vi "Main.vi"(11 "Module Admin":refnum<class "Delacor_lib_QMH_Module Admin.lvclass">) -> ()   [LabVIEW 2024, in "MQTTClient.lvlib"]
doc: "This template is based from the Queued Message Handler design pattern and the Queued Message Handler Project Template that ships with LabVIEW 2014.\n\nThe main difference is that the Queue is private to this module and communication between modules is done via Broadcast and Request events.\n\nRequest events are wrapped via public API methods and are handled in the Event handler loop in this VI.\nAny module can register for Broadcast events sent by this module.\n\nThe Event Handling Loop generates messages based on user interface actions.\n\nThe Message Handling Loop processes messages generated by the Event Handling Loop, or by other messages. The messages are string values, so new messages can be added easily to the Message Cases case structure in the Message Handling Loop. Each message cluster can also provide an optional value for Message Data, which is a variant that can be converted to whatever message-specific data is required.\n_____\nBased on Delacor QMH Project Template 3.1.0.34.\n\n<b>Note:</b> This VI was modified by the <b>Validate DQMH Module</b> tool to add a call to the Error Reported VI at the end of the 'Exit' MHL frame.\n\n<b>Note:</b> This VI was modified by the <b>Validate DQMH Module</b> tool to call the Release Message Queue VI in the top-level Error case.\n\n<b>Note:</b> This VI was modified by the <b>Validate DQMH Module</b> tool to wrap the FP.Open method in the module close code with a Conditional Disable Structure so it does not execute when the Main VI is running as a built EXE."
uses:
  MQTTClient.lvlib
  <vilib>/Delacor/Delacor QMH/Libraries/Module Admin_class/Delacor_lib_QMH_Module Admin.lvclass
  <vilib>/MGI/Panel Manager/Panel/Panel/Panel.lvclass
  <vilib>/Utility/miscctls.llb/LVPointTypeDef.ctl
  <vilib>/LabVIEW Open Source Project/MQTT Connection/MQTT_Base/Base Class/Public Events -- cluster.ctl
  <vilib>/LabVIEW Open Source Project/MQTT Control Packets/Control Packets/PUBLISH/PUBLISH.lvclass
  C:/Program Files/National Instruments/LabVIEW 2025/vi.lib/LabVIEW Open Source Project/MQTT Control Packets/Control Packets/ControlPacket/ControlPacket.lvclass
  <vilib>/LabVIEW Open Source Project/MQTT Client/Client class/Public Events -- cluster.ctl
  <vilib>/LabVIEW Open Source Project/MQTT Control Packets/Control Packets/CONNACK/Connect Return Code -- enum.ctl
  Module Data--cluster.ctl
  <vilib>/LabVIEW Open Source Project/MQTT Client/Client class/Client.lvclass
  C:/Program Files/National Instruments/LabVIEW 2025/vi.lib/LabVIEW Open Source Project/MQTT Connection/MQTT_Base/Base Class/MQTT_Base.lvclass
  MQTT Configuration--cluster.ctl
  <vilib>/Delacor/Delacor QMH/Libraries/Message Queue_class/Delacor_lib_QMH_Message Queue.lvclass/Delacor_lib_QMH_Message Queue.ctl
  Stop Argument--cluster.ctl
  <vilib>/Delacor/Delacor QMH/Libraries/Module Admin_class/Delacor_lib_QMH_Module Admin.lvclass/Delacor_lib_QMH_Module Admin.ctl
  Initialise Connection Argument--cluster.ctl
  Ping Connection Argument--cluster.ctl
  Publish to MQTT Topic Argument--cluster.ctl
  Close Connection Argument--cluster.ctl
  Connect to MQTT Server Argument--cluster.ctl
  Sleep Ping Helper Loop Argument--cluster.ctl
  Subscribe to MQTT Topic Argument--cluster.ctl
  Launch Argument--cluster.ctl
  <vilib>/LabVIEW Open Source Project/MQTT Control Packets/Control Packets/ControlPacket/ControlPacket.lvclass/ControlPacket.ctl
  <vilib>/Delacor/Delacor QMH/Libraries/Message Queue_class/Delacor_lib_QMH_Enqueue Message (Single).vi
  <vilib>/Delacor/Delacor QMH/Libraries/Module Admin_class/Delacor_lib_QMH_Get External Launch.vi
  <vilib>/Utility/error.llb/Error Cluster From Error Code.vi
  <vilib>/ErrorRing/Error Ring.xnode
  <vilib>/Delacor/Delacor QMH/Libraries/Message Queue_class/Delacor_lib_QMH_Message Queue.lvclass
  <vilib>/MGI/Panel Manager/Panel/Panel Helper/Panel Helper.lvclass
  <vilib>/LabVIEW Open Source Project/MQTT Connection/MQTT_Base/Base Class/MQTT_Base.lvclass
  <vilib>/LabVIEW Open Source Project/MQTT Control Packets/Control Packets/ControlPacket/ControlPacket.lvclass
  <vilib>/LabVIEW Open Source Project/MQTT Control Packets/Control Packets/CONNACK/CONNACK.lvclass
panel:
  out "Published":bool
  out "connected":bool
  out "Server responded":bool
  in  "Panel":refnum<class "Panel.lvclass">
  in  "Simulate MHL Error":bool
  in  "Simulate EHL Error":bool
  out "error out":errorcluster
  out "Status":string
  # "This is a template that creates a DQMH Singleton using the MGI Panel Manager Framwork.\n\nImplement your user interface on this front panel. The Panel Manager Framework will manage showing and hiding the panel in the appropriate spot. \n\nSee the block diagram for more information on how to use this template."
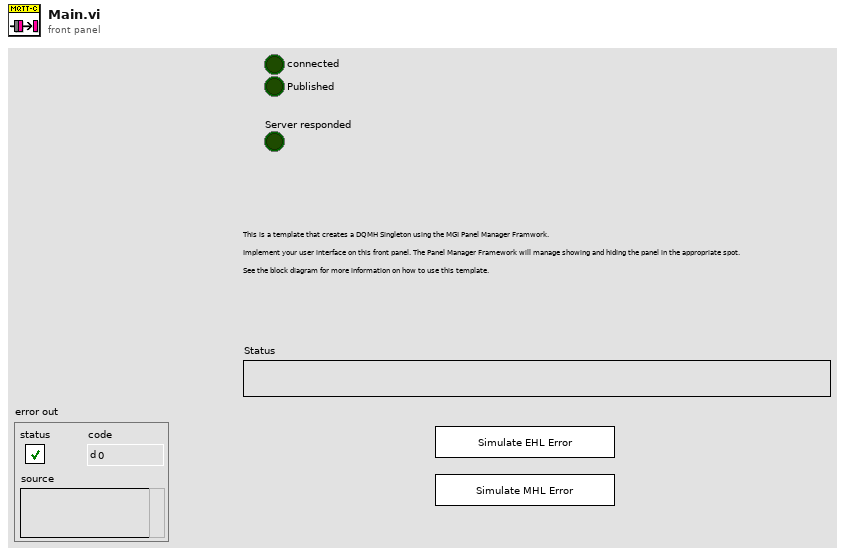
[diagram p1: front panel]
types:
  T1 = typedef "MQTT Client.lvlib/Client.lvclass/Public Events -- cluster.ctl" = cluster{"Connection Status":refnum<user-event>, "Connected":refnum<user-event>, "Application Message":refnum<user-event>}
  T2 = typedef "MQTT Base.lvlib/MQTT_Base.lvclass/Public Events -- cluster.ctl" = cluster{"Stop Event":refnum<user-event>, "Error Event":refnum<user-event>, "Inbound Message":refnum<user-event>}
  T3 = typedef "LVPointTypeDef.ctl" = cluster{"Horizontal":i16, "Vertical":i16}
  T4 = typedef "MQTTClient.lvlib/Request Events--cluster.ctl" = cluster{"Stop Module":refnum<user-event>, "Show Panel":refnum<user-event>, "Hide Panel":refnum<user-event>, "Get Module Execution Status":refnum<user-event>, "Show Diagram":refnum<user-event>, "Change Panel":refnum<user-event>, "Initialise Connection":refnum<user-event>, "Ping Connection":refnum<user-event>, "Publish to MQTT Topic":refnum<user-event>, "Close Connection":refnum<user-event>, "Connect to MQTT Server":refnum<user-event>, "Private":cluster{"Reset Ping Helper Loop Timeout":refnum<user-event>, "Sleep Ping Helper Loop":refnum<user-event>, "Register MQTT Client Events":refnum<user-event>}, "Subscribe to MQTT Topic":refnum<user-event>, "Launch":refnum<user-event>, "Private.Wake Connection Helper Loop":refnum<user-event>}
  T5 = typedef "Panel.lvlib/Panel Helper.lvclass/Panel Events.ctl" = cluster{"My Panel":refnum<user-event>, "Top Level Initialized":refnum<user-event>}
  T6 = typedef "MQTTClient.lvlib/Module Data--cluster.ctl" = cluster{"Status":string, "MQTT_Base":refnum<class "Client.lvclass">, "Published Values":map{string, string}, "Configuration":T7, "Subscribed Values":map{string, string}}
  T7 = typedef "MQTTClient.lvlib/MQTT Configuration--cluster.ctl" = cluster{"Client-ID":string, "Server Address":string, "Server Port":u16}
  T8 = typedef "MQTTClient.lvlib/Stop Argument--cluster.ctl" = cluster{"Origin":string, "Exit via Stop Module Req?":bool, "Wait for Module to stop?":bool}
  T9 = typedef "MQTTClient.lvlib/Initialise Connection Argument--cluster.ctl" = cluster{"Client ID":string, "Server Address":string, "Server Port":u16}
  T10 = typedef "MQTTClient.lvlib/Ping Connection Argument--cluster.ctl" = cluster{"Boolean":bool}
  T11 = typedef "MQTTClient.lvlib/Publish to MQTT Topic Argument--cluster.ctl" = cluster{"Topic":string, "Value":string}
  T12 = typedef "MQTTClient.lvlib/Close Connection Argument--cluster.ctl" = cluster{"Boolean":bool}
  T13 = typedef "MQTTClient.lvlib/Connect to MQTT Server Argument--cluster.ctl" = cluster{"Boolean":bool}
  T14 = typedef "MQTTClient.lvlib/Sleep Ping Helper Loop Argument--cluster.ctl" = cluster{"Boolean":bool}
  T15 = typedef "MQTTClient.lvlib/Subscribe to MQTT Topic Argument--cluster.ctl" = cluster{"Topic":string}
  T16 = typedef "MQTTClient.lvlib/Launch Argument--cluster.ctl" = cluster{"Boolean":bool}
  T17 = enum32{"invalid lock state", "Not Locked", "Locked (No Password)", "Password-protected"}
  T18 = typedef "MQTTClient.lvlib/Config--cluster.ctl" = cluster{"Client-ID":string, "Server Address":string, "Server Port":u16}
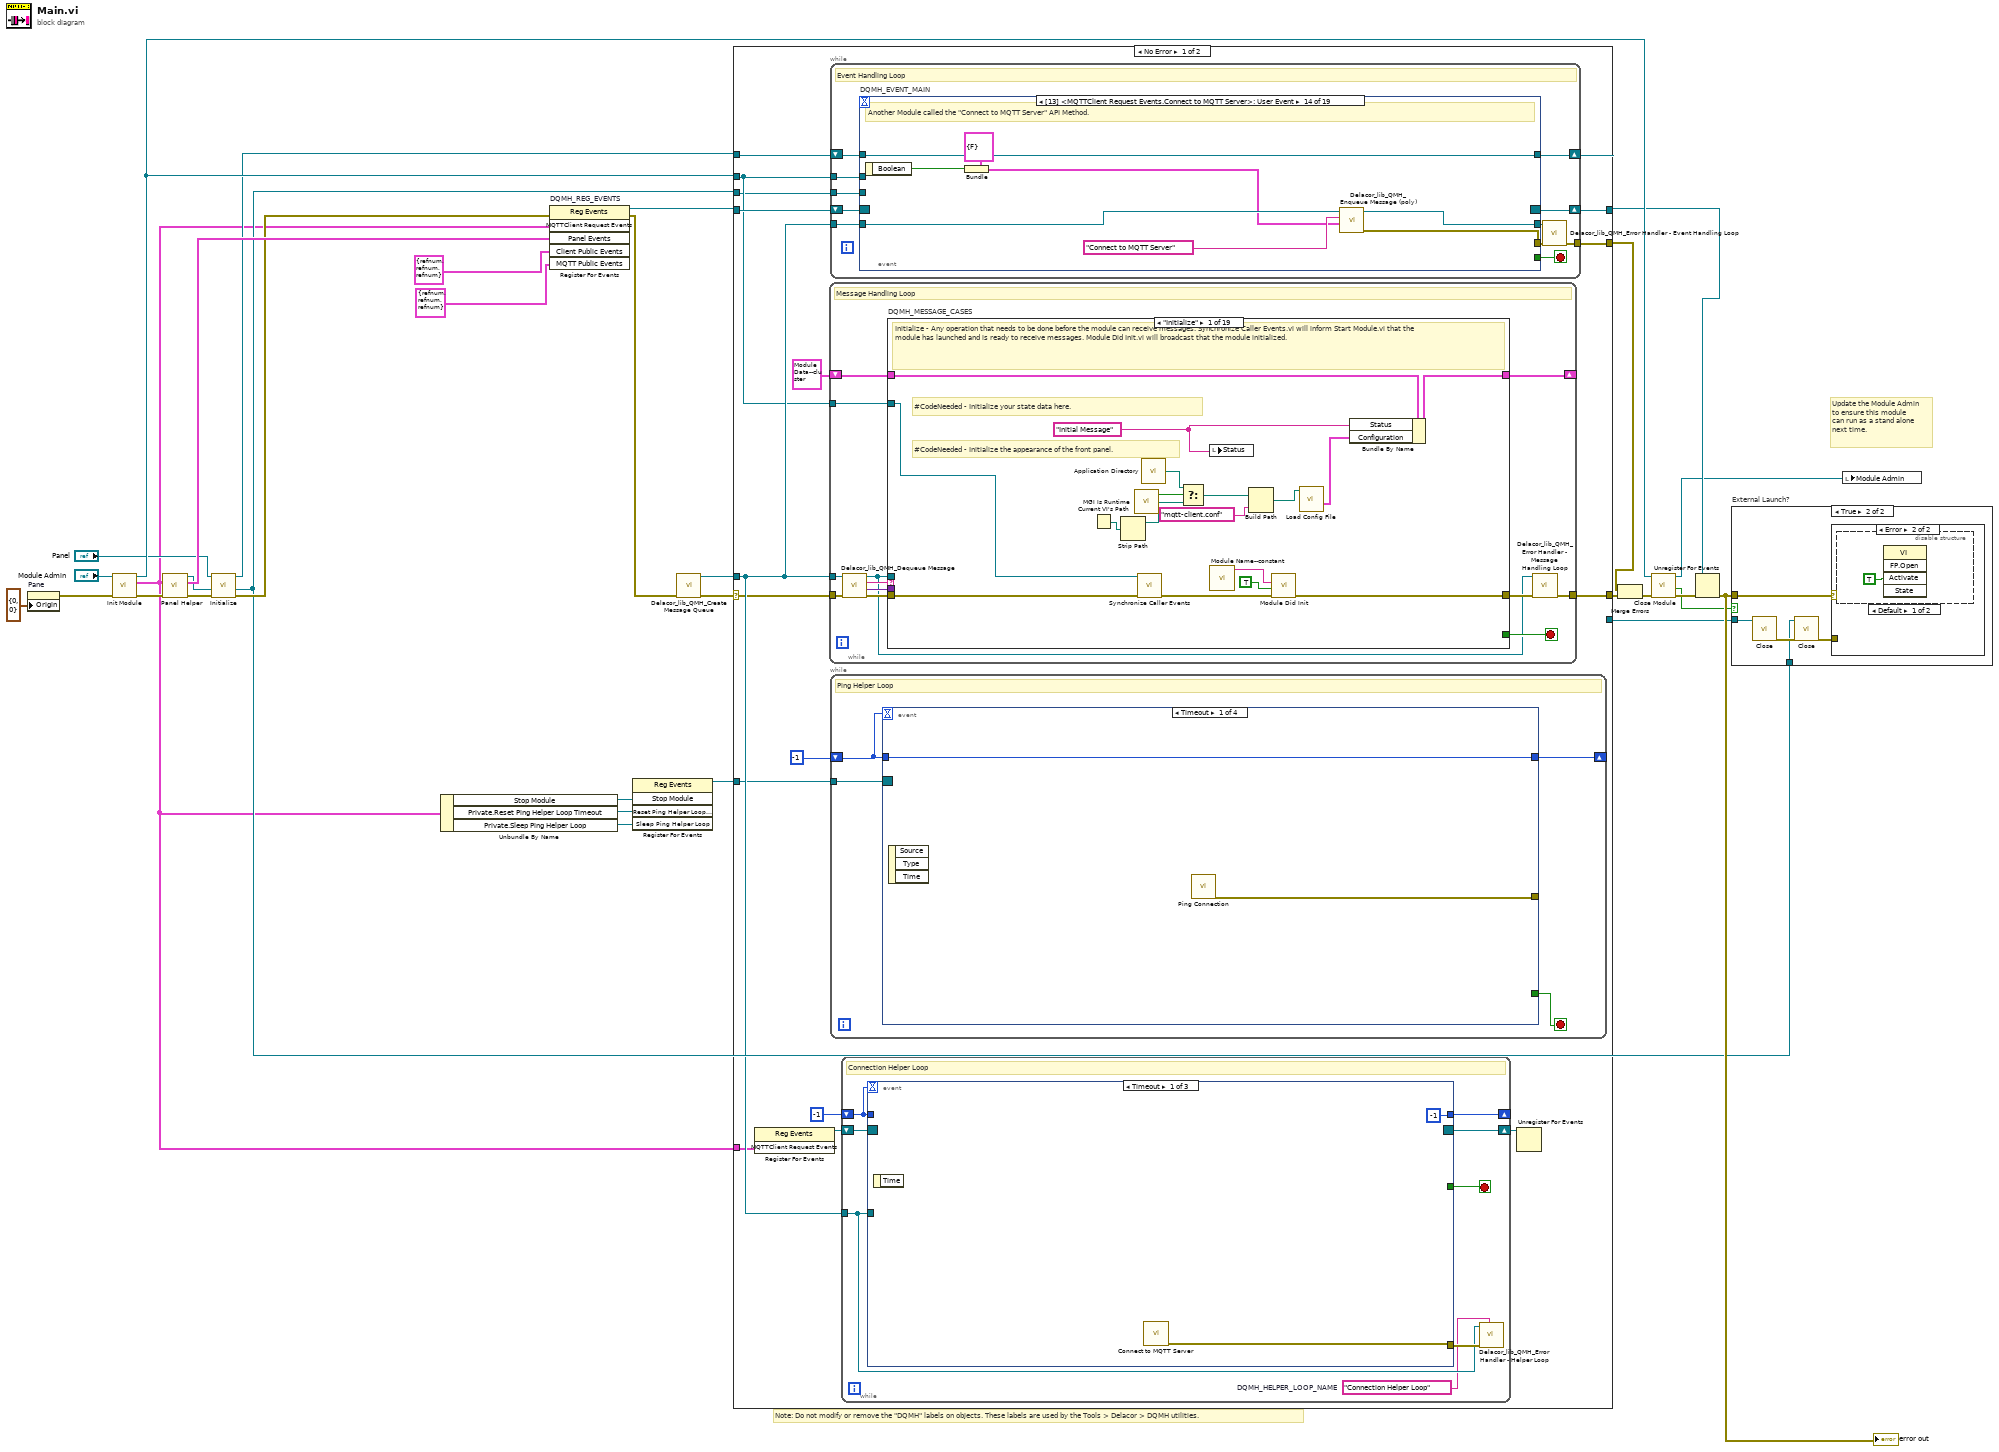
[diagram p0: block diagram]
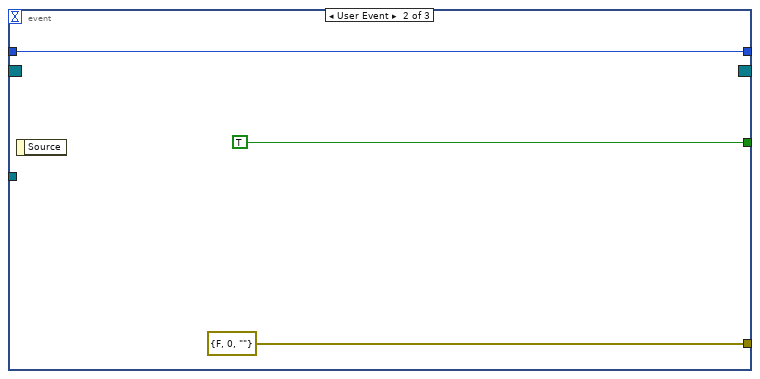
[diagram p5: hidden frame]
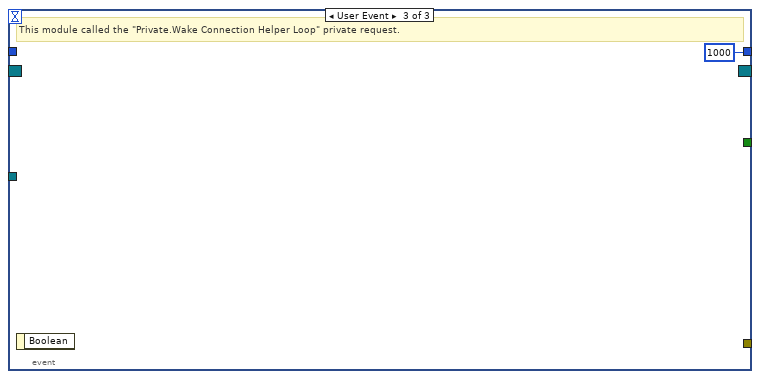
[diagram p6: hidden frame]
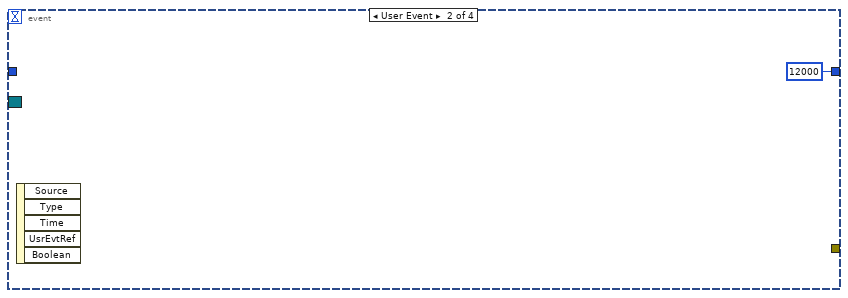
[diagram p7: hidden frame]
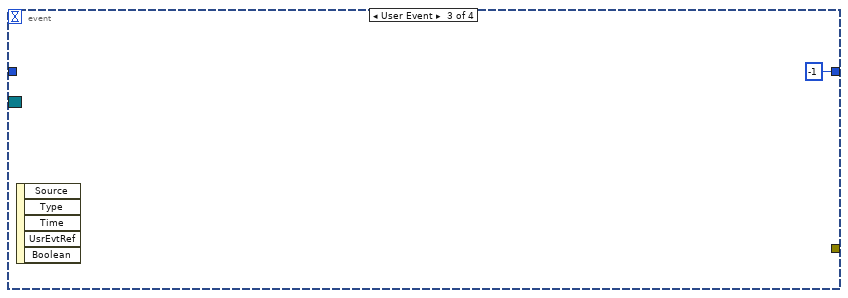
[diagram p8: hidden frame]
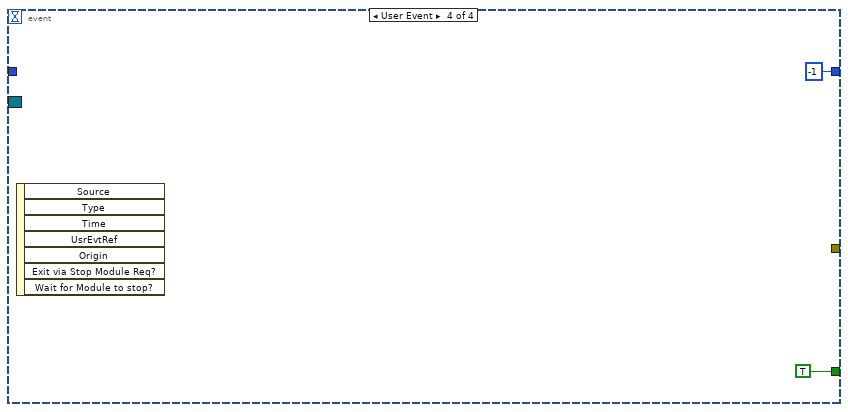
[diagram p9: hidden frame]
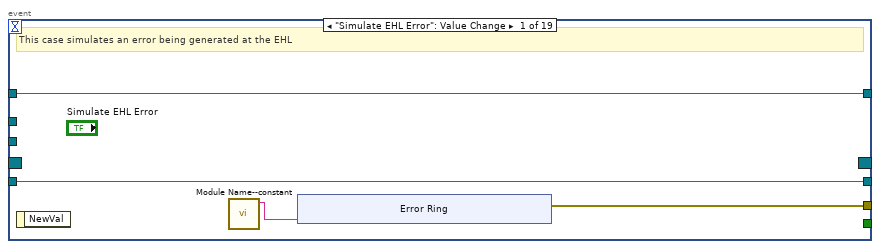
[diagram p10: hidden frame]
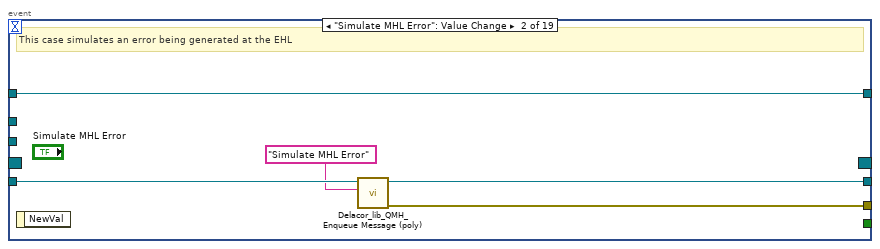
[diagram p11: hidden frame]
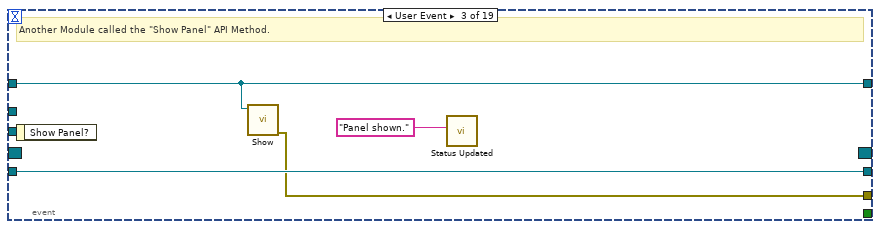
[diagram p12: hidden frame]
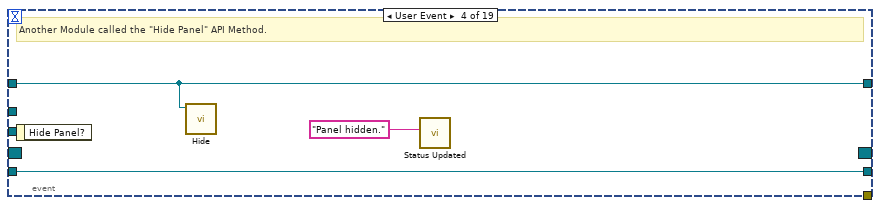
[diagram p13: hidden frame]
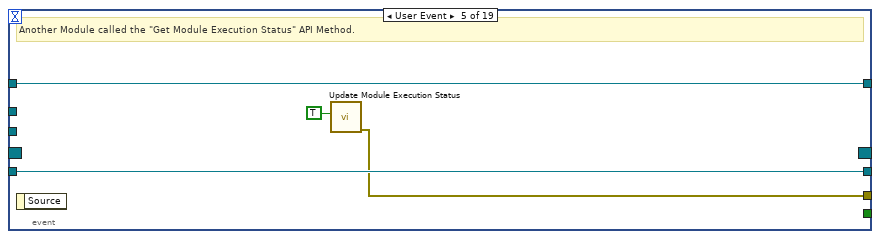
[diagram p14: hidden frame]
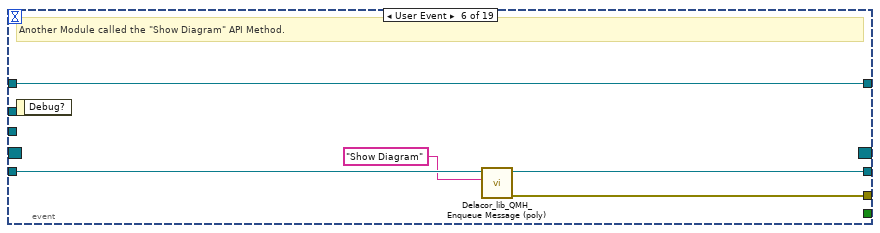
[diagram p15: hidden frame]
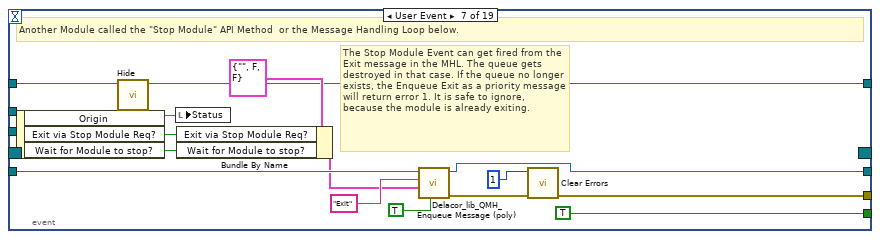
[diagram p16: hidden frame]
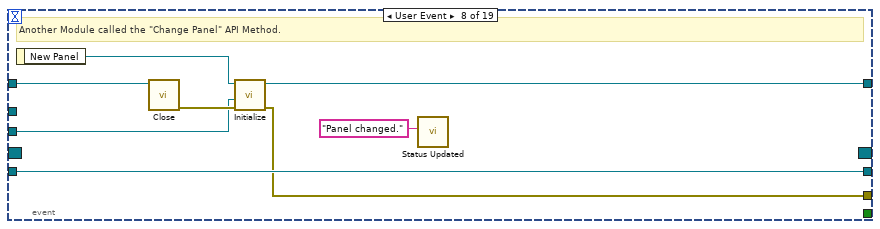
[diagram p17: hidden frame]
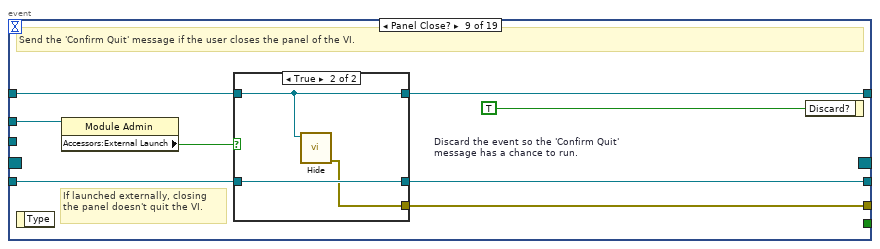
[diagram p18: hidden frame]
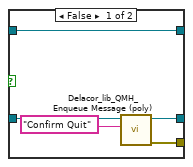
[diagram p19: hidden frame]
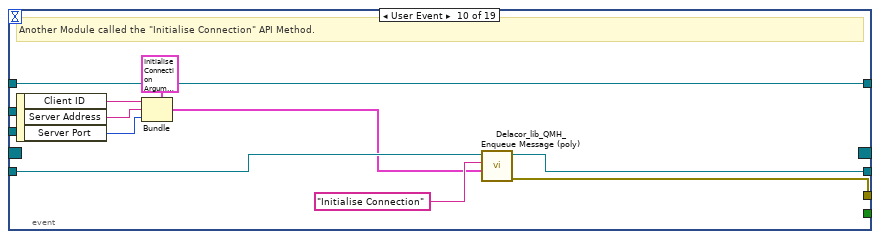
[diagram p20: hidden frame]
diagram:
  # "Note: Do not modify or remove the \"DQMH\" labels on objects. These labels are used by the Tools > Delacor > DQMH utilities."
  # "Update the Module Admin to ensure this module can run as a stand alone next time."
  n1 = property on="Pane" class="Pane"("Origin"=T3 {"Horizontal"=0, "Vertical"=0}) -> (error out=w8:errorcluster)  [unwired: 2 in, 1 out]
  n2 = call "Init Module.vi"("error in (no error)"=w8, "Singleton Module Admin in"="Module Admin") -> ("error out"=w18:errorcluster, "MQTTClient Request Events"=w1:T4, "Singleton Module Admin out"=w32:refnum<class "Delacor_lib_QMH_Module Admin.lvclass">)  [unwired: 7 in]
  n3 = call <vilib>:"Panel Helper.vi"("Error In"=w18) -> ("Error Out"=w15:errorcluster, "Panel Events"=w17:T5, "Panel Helper out"=w14:refnum<class "Panel Helper.lvclass">)  [unwired: 8 in]
  n4 = call <vilib>:"Initialize.vi"("error in (no error)"=w15, "My Helper in"=w14, "Panel In"="Panel") -> ("error out"=w12:errorcluster, "My Helper out"=w11:refnum<class "Panel Helper.lvclass">, "Panel Out"=w10:refnum<class "Panel.lvclass">)  [unwired: 6 in]
  n5 = Unbundle By Name(w1) -> ("Stop Module"=w5:refnum<user-event>, "Private.Reset Ping Helper Loop Timeout"=w6:refnum<user-event>, "Private.Sleep Ping Helper Loop"=w7:refnum<user-event>)
  n6 = register-events "DQMH_REG_EVENTS"(error in=w12, w1, w17, T1 {"Connection Status"=refnum, "Connected"=refnum, "Application Message"=refnum} ("Client Public Events"), T2 {"Stop Event"=refnum, "Error Event"=refnum, "Inbound Message"=refnum} ("MQTT Public Events")) -> (reference out=w29:refnum<event-registration>, error out=w16:errorcluster)  [unwired: 1 in]
  n7 = register-events(w5, w6, w7) -> (reference out=w4:refnum<event-registration>)  [unwired: 2 in, 1 out]
  n8 = call <vilib>:"Delacor_lib_QMH_Create Message Queue.vi"("error in"=w16) -> ("error out"=w20:errorcluster, "Message Queue"=w28:refnum<class "Delacor_lib_QMH_Message Queue.lvclass">)  [unwired: 9 in]
  n9 = case shown="No Error" w20 {
    selector: w20 -> [w43 w511]
    tunnel: [w49 w511] -> w31
    tunnel: [w48 w516] -> w30
    tunnel: w29 -> [w46 w516]
    tunnel: w28 -> [w45 w507]
    tunnel: [w44 _] -> w24
    tunnel: w32 -> [w42 w512]
    tunnel: w10 -> [w40 w508]
    tunnel: w11 -> [w41 _]
    tunnel: [w39 w508] -> w19
    tunnel: w4 -> [w38 _]
    tunnel: w1 -> [w36 _]
    frame No Error {
      n10 = register-events ("DQMH_HELPER_REGFOREVENTS")(w36) -> (reference out=w34:refnum<event-registration>)  [unwired: 2 in, 1 out]
      n11 = while {
        tunnel: w45 -> [w237]
        shift-right: [w243] -> _
        shift-left: T6 {"Status"="", "MQTT_Base"=refnum, "Published Values"={}, "Configuration"={"Client-ID"="", "Server Address"="", "Server Port"=0}, "Subscribed Values"={}} ("Data Cluster") -> [w244]
        tunnel: w43 -> [w241]
        tunnel: [w235] -> w49
        tunnel: w42 -> [w234]
        stop <- w242 stop-if-true
        # "Message Handling Loop"
        n12 = call-dynamic "Delacor_lib_QMH_Dequeue Message.vi"("error in"=w241, "Message Queue in"=w237) -> ("error out"=w240:errorcluster, "Message Data"=w238:variant, "Message"=w239:string, "Message Queue out"=w236:refnum<class "Delacor_lib_QMH_Message Queue.lvclass">)  [unwired: 6 in]
        n13 = case "DQMH_MESSAGE_CASES" shown="\"Initialize\"" w239 {
          selector: w239 -> [_ _ _ _ _ _ _ _ _ _ _ _ _ _ _ _ _ _ w496]
          tunnel: w236 -> [_ _ _ _ _ _ _ _ _ _ _ _ _ _ _ w460 w475 w492 _]
          tunnel: w240 -> [w256 w268 w272 w290 w306 w320 w358 w380 w400 w415 w428 w438 w441 w444 w449 w466 w479 w494 _]
          tunnel: [w257 w269 w271 w288 w298 w308 w349 w376 w390 w403 w425 w435 w439 w442 w447 w457 w477 w488 w497] -> w245
          tunnel: w244 -> [w262 w270 w273 w289 w292 w312 w354 w369 w394 w407 w417 w432 w440 w443 w448 w465 w478 w491 w498]
          tunnel: [w261 w270 w273 w289 w302 w311 w353 w368 w393 w406 w416 w432 w440 w443 w448 w465 w478 w491 w498] -> w243
          tunnel: [_ _ _ _ _ _ _ _ _ _ _ _ _ _ _ _ _ w490 _] -> w242
          tunnel: w238 -> [_ w267 _ _ w305 w319 w357 w379 w399 w413 w427 w437 _ _ _ w464 _ w487 _]
          tunnel: w234 -> [w254 _ _ _ _ _ _ _ _ _ _ _ _ _ _ w459 _ w481 _]
          frame "Initialize" {
            w260 = "Initial Message" ("Initial Message")
            # "#CodeNeeded - Initialize the appearance of the front panel."
            # "#CodeNeeded - Initialize your state data here."
            # "Initialize - Any operation that needs to be done before the module can receive messages. Synchronize Caller Events.vi will inform Start Module.vi that the module has launched and is ready to receive messages. Module Did Init.vi will broadcast that the module initialized."
            n14 = Current VI's Path() -> (path=w247:path)
            n15 = Strip Path(path=w247) -> (stripped path=w246:path)  [unwired: 1 out]
            n16 = call <userlib>:"MGI Is Runtime.vi"() -> ("Run Time System?"=w250:bool)  [unwired: 7 in]
            n17 = call "Synchronize Caller Events.vi"("error in (no error)"=w256, "Singleton Module Admin in"=w254) -> ("error out"=w255:errorcluster)  [unwired: 8 in, 1 out]
            n18 = call <vilib>:"Application Directory.vi"() -> ("Application Directory"=w249:path)
            n19 = Select(t=w249, s=w250, f=w246) -> (s? t:f=w248:path)
            n20 = local write "Status"(w260) -> ()
            n21 = call "Module Name--constant.vi"() -> ("Module Name"=w258:string)  [unwired: 11 in]
            n22 = Build Path(base path=w248, name or relative path="mqtt-client.conf") -> (appended path=w252:path)
            n23 = call "Module Did Init.vi"("error in (no error)"=w255, "Initialized?"=TRUE, "Origin"=w258) -> ("error out"=w257:errorcluster)  [unwired: 8 in]
            n24 = call "Load Config File.vi"("File Path"=w252) -> ("value"=w251:T18)  [unwired: 10 in]
            n25 = Bundle By Name(cluster=w262, "Status"=w260, "Configuration"=w251) -> (w261:T6)
          }
          frame "Update Display" {
            # "Broadcast updated status to any VI registered to listen to this module's broadcast events."
            # "Convert the message data to a string to display in the Status indicator."
            # "#CodeRecommended - If you wish to decouple the Message Handling Loop from your user interface, consider creating User Events (like the \"Stop\" event in this VI) to message the Event Handling Loop whenever the user interface needs updating."
            # "Update Display - Update user interface here."
            n26 = Variant To Data(error in=w268, type="" ("Empty String Constant"), Variant=w267) -> (data=w265:string, error out=w264:errorcluster)
            "Status" <- w265
            n27 = call "Status Updated.vi"("error in (no error)"=w264, "Status"=w265) -> ("error out"=w263:errorcluster)  [unwired: 9 in]
            n28 = Merge Errors(w263) -> (w269:errorcluster)
          }
          frame "Show Diagram" {
            # "Show Diagram - Show the block diagram of this VI. Used as a debugging tool. There is a button in the module tester that fires the Show Diagram request, which runs this message. Note that the diagram will not be displayed if it is password-protected and the password is not in the cache."
            n29 = disable-structure shown="RUN_TIME_ENGINE==False" {
              disable-tunnel: [w281 w287] -> w271
              disable-tunnel: w272 -> [w280 w287]
              frame condition #0 (active) {
                # "functionality not available in exe"
                n30 = invoke class="VI" method="Lock State.Get"(error in=w280) -> (error out=w279:errorcluster, "Get Lock State"=w278:T17, "pwd in cache"=w275:bool)  [unwired: 3 in, 1 out]
                n31 = Equal?(x=T17."Password-protected", y=w278) -> (x = y?=w276:bool)
                n32 = Compound Arithmetic op=AND(w276, invert w275) -> (w274:bool)
                n33 = case shown="False" w274 {
                  tunnel: [w284 w286] -> w281
                  tunnel: w279 -> [w282 w286]
                  frame False {
                    n34 = property class="VI"(error in=w282, "BDWin.Open"=TRUE ("Block Diagram Window:Open")) -> (error out=w284:errorcluster)  [unwired: 1 in, 1 out]
                    n35 = call "Status Updated.vi"("Status"="Block Diagram shown." ("format string")) -> ()  [unwired: 10 in, 1 out]
                  }
                  frame True {
                    # "Password-protected VI, and the password is not in the cache. Do not show the diagram."
                  }
                }
              }
              frame condition #1 {
              }
            }
          }
          frame "--- Module Specific ---" {
            # "Separator -- The following cases handle messages specific to this Module."
            n36 = Merge Errors(w290) -> (w288:errorcluster)
          }
          frame "Initialise Connection" {
            # "Initialises a connection to the MQTT broker."
            n37 = Variant To Data(error in=w306, type=T9 {"Client ID"="BTSCLIENT-001", "Server Address"="localhost", "Server Port"=1883} ("Initialise Connection Argument"), Variant=w305) -> (data=w303:T9)  [unwired: 1 out]
            n38 = Unbundle By Name(w292) -> ("MQTT_Base"=w296:refnum<class "Client.lvclass">)
            n39 = Unbundle By Name(w303) -> ("Client ID"=w301:string, "Server Address"=w299:string, "Server Port"=w300:u16)
            n40 = call <vilib>:"Stop.vi"("MQTT_Base in"=w296) -> ("error out"=w294:errorcluster, "MQTT_Base out"=w295:refnum<class "Client.lvclass">)  [unwired: 8 in, 1 out]
            n41 = call <vilib>:"Destroy.vi"("error in (no error)"=w294, "MQTT_Base in"=w295) -> ("error out"=w293:errorcluster)  [unwired: 8 in, 1 out]
            n42 = call <vilib>:"Clear Errors.vi"("error in (no error)"=w293) -> ("error out"=w291:errorcluster)  [unwired: 5 in, 1 out]
            n43 = call "Initialise Connection--SubVI.vi"("Client ID"=w301, "error in (no error)"=w291, "remote port (1883)"=w300, "address (localhost)"=w299) -> ("error out"=w298:errorcluster, "MQTT_Base out"=w297:refnum<class "Client.lvclass">)  [unwired: 6 in]
            n44 = Bundle By Name(cluster=w292, "Configuration.Client-ID"=w301, "Configuration.Server Address"=w299, "Configuration.Server Port"=w300, "MQTT_Base"=w297) -> (w302:T6)
          }
          frame "Connect to MQTT Server" {
            # "Connects to MQTT server."
            n45 = Variant To Data(error in=w320, type=T13 {"Boolean"=FALSE} ("Connect to MQTT Server Argument"), Variant=w319) -> (error out=w310:errorcluster)  [unwired: 1 out]
            n46 = Unbundle By Name(w312) -> ("MQTT_Base"=w315:refnum<class "Client.lvclass">)
            n47 = call <vilib>:"isConnected.vi"("error in (no error)"=w310, "Client in"=w315) -> ("error out"=w317:errorcluster, "connected"=w313:bool, "Client out"=w316:refnum<class "Client.lvclass">)  [unwired: 7 in]
            n48 = case shown="False" w313 {
              selector: w313 -> [_ w345]
              tunnel: w317 -> [w336 w346]
              tunnel: w316 -> [w335 w347]
              tunnel: [w330 w346] -> w309
              tunnel: [w333 w347] -> w314
              tunnel: [w331 w345] -> w307
              frame False {
                # "Connect"
                n49 = call <vilib>:"Connect to Server.vi"("timeout (2000 ms)"=2000, "Keep Alive (s)"=u16 60, "error in (no error)"=w336, "Client in"=w335) -> ("error out"=w332:errorcluster, "timed out"=w328:bool, "Client out"=w334:refnum<class "Client.lvclass">)  [unwired: 4 in, 1 out]
                n50 = case shown="True" w328 {
                  tunnel: w334 -> [w341 w344]
                  tunnel: [w340 w344] -> w333
                  tunnel: w332 -> [w339 w343]
                  tunnel: [w338 FALSE ("connected")] -> w331
                  tunnel: [w337 w343] -> w330
                  frame False {
                    n51 = call <vilib>:"isConnected.vi"("error in (no error)"=w339, "Client in"=w341) -> ("error out"=w337:errorcluster, "connected"=w338:bool, "Client out"=w340:refnum<class "Client.lvclass">)  [unwired: 7 in]
                  }
                  frame True {
                  }
                }
              }
              frame True {
                # "Already Connected"
              }
            }
            "connected" <- w307
            n52 = Bundle By Name(cluster=w312, "MQTT_Base"=w314) -> (w311:T6)
            n53 = case shown="False" w307 {
              tunnel: w309 -> [w322 w326]
              tunnel: [w321 w324] -> w308
              frame False {
                n54 = call "Wake Connection Helper Loop.vi"() -> ("error out"=w323:errorcluster)  [unwired: 11 in]
                n55 = Merge Errors(w323, w322) -> (w321:errorcluster)
              }
              frame True {
                n56 = call "Reset Ping Helper Loop Timeout.vi"() -> ("error out"=w325:errorcluster)  [unwired: 11 in]
                n57 = Merge Errors(w325, w326) -> (w324:errorcluster)
              }
            }
          }
          frame "Ping Connection" {
            # "Pings the MQTT broker."
            n58 = Variant To Data(error in=w358, type=T10 {"Boolean"=FALSE} ("Ping Connection Argument"), Variant=w357) -> (error out=w351:errorcluster)  [unwired: 1 out]
            n59 = Unbundle By Name(w354) -> ("MQTT_Base"=w355:refnum<class "Client.lvclass">)
            n60 = call <vilib>:"Ping.vi"("error in (no error)"=w351, "Client in"=w355) -> ("error out"=w350:errorcluster, "Server responded"=w348:bool, "Client out"=w352:refnum<class "Client.lvclass">)  [unwired: 6 in, 1 out]
            "Server responded" <- w348
            n61 = Bundle By Name(cluster=w354, "MQTT_Base"=w352) -> (w353:T6)
            n62 = case shown="False" w348 {
              tunnel: w350 -> [w360 w363]
              tunnel: [w359 w362] -> w349
              frame False {
                n63 = call "Wake Connection Helper Loop.vi"() -> ("error out"=w361:errorcluster)  [unwired: 11 in]
                n64 = Merge Errors(w361, w360) -> (w359:errorcluster)
              }
              frame True {
                n65 = call "Reset Ping Helper Loop Timeout.vi"() -> ("error out"=w364:errorcluster)  [unwired: 11 in]
                n66 = Merge Errors(w364, w363) -> (w362:errorcluster)
              }
            }
          }
          frame "Publish to MQTT Topic" {
            # "Publishes to a MQTT topic."
            n67 = Variant To Data(error in=w380, type=T11 {"Topic"="", "Value"=""} ("Publish to MQTT Topic Argument"), Variant=w379) -> (data=w377:T11, error out=w366:errorcluster)
            n68 = Unbundle By Name(w377) -> ("Topic"=w370:string, "Value"=w367:string)
            n69 = String To Byte Array(string=w367) -> (unsigned byte array=w373:u8[])
            n70 = Unbundle By Name(w369) -> ("MQTT_Base"=w375:refnum<class "Client.lvclass">)
            n71 = call <vilib>:"Publish (Raw Payload).vi"("error in (no error)"=w366, "Binary Payload"=w373, "Topic Name"=w370, "Client in"=w375) -> ("error out"=w365:errorcluster, "Published"=w371:bool, "Client out"=w374:refnum<class "Client.lvclass">)  [unwired: 5 in]
            "Published" <- w371
            n72 = Bundle By Name(cluster=w369, "MQTT_Base"=w374) -> (w372:T6)
            n73 = case shown="True" w371 {
              tunnel: w372 -> [w386 w389]
              tunnel: w370 -> [w387 _]
              tunnel: [w384 w389] -> w368
              frame False {
                # "If publish fails remove record of last published value"
                n74 = Unbundle By Name(w386) -> ("Published Values"=w388:map{string, string})
                n75 = Remove From Map(10:w387, 11:w388) -> (3:w385:map{string, string})  [unwired: 2 out]
                n76 = Bundle By Name(cluster=w386, "Published Values"=w385) -> (w384:T6)
              }
              frame True {
              }
            }
            n77 = flat-sequence {
              tunnel: [w382] -> w376
              tunnel: w365 -> [w381]
              frame #0 {
                n78 = call "Reset Ping Helper Loop Timeout.vi"() -> ("error out"=w383:errorcluster)  [unwired: 11 in]
                n79 = Merge Errors(w383, w381) -> (w382:errorcluster)
              }
            }
          }
          frame "Subscribe to MQTT Topic" {
            # "Subscribes to an MQTT topic."
            n80 = Variant To Data(error in=w400, type=T15 {"Topic"=""} ("Subscribe to MQTT Topic Argument"), Variant=w399) -> (data=w397:T15, error out=w391:errorcluster)
            n81 = Unbundle By Name(w397) -> ("Topic"=w396:string)
            n82 = Unbundle By Name(w394) -> ("MQTT_Base"=w395:refnum<class "Client.lvclass">)
            n83 = call <vilib>:"Subscribe (Scalar).vi"("error in (no error)"=w391, "Topic Filter"=w396, "Client in"=w395) -> ("error out"=w390:errorcluster, "Client out"=w392:refnum<class "Client.lvclass">)  [unwired: 6 in, 1 out]
            n84 = Bundle By Name(cluster=w394, "MQTT_Base"=w392) -> (w393:T6)
          }
          frame "Handle PUBLISH Data" {
            n85 = Variant To Data(error in=w415, type=refnum<class "PUBLISH.lvclass"> refnum ("PUBLISH"), Variant=w413) -> (data=w410:refnum<class "PUBLISH.lvclass">, error out=w411:errorcluster)
            n86 = Unbundle By Name(w407) -> ("Subscribed Values"=w408:map{string, string})
            n87 = call <vilib>:"getTopicName.vi"("error in (no error)"=w411, "PUBLISH in"=w410) -> ("error out"=w404:errorcluster, "Topic"=w402:string, "PUBLISH out"=w409:refnum<class "PUBLISH.lvclass">)  [unwired: 7 in]
            n88 = call <vilib>:"Read Payload.vi"("ControlPacket in"=w409) -> ("Payload"=w412:u8[])  [unwired: 9 in, 1 out]
            n89 = Byte Array To String(unsigned byte array=w412) -> (string=w401:string)
            n90 = Insert Into Map(map in=w408, key=w402, value=w401) -> (map out=w405:map{string, string})  [unwired: 2 out]
            n91 = Bundle By Name(cluster=w407, "Subscribed Values"=w405) -> (w406:T6)
            n92 = call "Broadcast MQTT Topic and Value.vi"("error in"=w404, "Value"=w401, "Topic"=w402) -> ("error out"=w403:errorcluster)  [unwired: 8 in]
          }
          frame "Close Connection" {
            # "Closes the MQTT connection."
            n93 = Variant To Data(error in=w428, type=T12 {"Boolean"=FALSE} ("Close Connection Argument"), Variant=w427) -> (error out=w419:errorcluster)  [unwired: 1 out]
            n94 = Unbundle By Name(w417) -> ("MQTT_Base"=w424:refnum<class "Client.lvclass">)
            n95 = call <vilib>:"Stop.vi"("error in (no error)"=w419, "MQTT_Base in"=w424) -> ("error out"=w422:errorcluster, "MQTT_Base out"=w423:refnum<class "Client.lvclass">)  [unwired: 7 in, 1 out]
            n96 = call <vilib>:"Destroy.vi"("error in (no error)"=w422, "MQTT_Base in"=w423) -> ("error out"=w420:errorcluster, "MQTT_Base out"=w421:refnum<class "Client.lvclass">)  [unwired: 8 in]
            n97 = call <vilib>:"Clear Errors.vi"("error in (no error)"=w420) -> ("error out"=w418:errorcluster)  [unwired: 5 in, 1 out]
            n98 = Bundle By Name(cluster=w417, "MQTT_Base"=w421) -> (w416:T6)
            n99 = call "Sleep Ping Helper Loop.vi"("error in"=w418) -> ("error out"=w425:errorcluster)  [unwired: 10 in]
          }
          frame "Launch" {
            # "Launches the MQTT Client based on configuration."
            n100 = Variant To Data(error in=w438, type=T16 {"Boolean"=FALSE} ("Launch Argument"), Variant=w437) -> (error out=w434:errorcluster)  [unwired: 1 out]
            n101 = Unbundle By Name(w432) -> ("Configuration.Client-ID"=w430:string, "Configuration.Server Address"=w429:string, "Configuration.Server Port"=w431:u16)
            n102 = call "Initialise Connection.vi"("Server Port"=w431, "error in"=w434, "Server Address"=w429, "Client ID"=w430) -> ("error out"=w433:errorcluster)  [unwired: 7 in]
            n103 = call "Connect to MQTT Server.vi"("error in"=w433) -> ("error out"=w435:errorcluster)  [unwired: 10 in]
          }
          frame "---Copy This Frame---" {
            # "Duplicate this frame when creating new messages.  Change this comment in the duplicated frame to describe this message."
            n104 = Merge Errors(w441) -> (w439:errorcluster)
          }
          frame "--- Exit and Error Handling---" {
            # "Separator - The following cases handle errors and exit messages."
            n105 = Merge Errors(w444) -> (w442:errorcluster)
          }
          frame "Simulate MHL Error" {
            # "Simulate an error occurring at the MHL"
            n106 = call "Module Name--constant.vi"() -> ("Module Name"=w446:string)  [unwired: 11 in]
            n107 = xnode "Error Ring"("parameter 0"=w446) -> ("error out"=w445:errorcluster)
            n108 = Merge Errors(w449, w445) -> (w447:errorcluster)
          }
          frame "Error" {
            # "#CodeRecommended - If you ever change the name of this \"Error\" message, you'll need to update the name in the Check Loop Error.vi as well."
            # "#CodeRecommended - If the module is running in standalone mode (External Launch = FALSE), this code will pop up an error dialog and call the 'Exit' message if an error occurs. Add more fine-grained error handling here."
            # "Error - Check the error message data and respond accordingly. This message is sent by the \"Error Handler\" VIs at the end of each loop in this application."
            n109 = property class="Module Admin"(reference=w459) -> ("Accessors:External Launch"=w458:bool)  [unwired: 1 in, 2 out]
            n110 = Variant To Data(error in=w466, type=errorcluster {"status"=FALSE, "code"=0, "source"=""} ("error constant"), Variant=w464) -> (data=w467:errorcluster, error out=w462:errorcluster)
            n111 = call "Error Reported.vi"("Error"=w467) -> ()  [unwired: 10 in, 1 out]
            n112 = case shown="True" w458 {
              tunnel: [w472 _] -> w461
              tunnel: w460 -> [w471 _]
              tunnel: w467 -> [w468 _]
              frame False {
                # "If the module is running standalone, then pop up an error dialog and call the \"Exit\" message."
                n113 = call <vilib>:"Simple Error Handler.vi"("error in (no error)"=w468) -> ()  [unwired: 4 in, 5 out]
                n114 = call-poly <vilib>:"Delacor_lib_QMH_Enqueue Message (poly).vi"("Priority Message? (F)"=TRUE, "Message"="Exit", "Message Queue in"=w471) -> ("error out"=w472:errorcluster)  [unwired: 7 in, 1 out]
              }
              frame True {
                # "If the module was launched externally, calling the Error Reported broadcast VI is the only action performed by the \"Error\" message. The module's caller can then process the error appropriately."
              }
            }
            n115 = Merge Errors(w462, w461) -> (w457:errorcluster)
            n116 = local write "error out"(w457) -> ()
          }
          frame "Confirm Quit" {
            # "#CodeNeeded - If you want to provide an \"Are you sure\" dialog (or some other notification) before the application exits, place that code here. This message is typically sent from a Panel Close? event."
            # "Confirm Quit - Message that can confirm whether or not the user wants to exit the application."
            n117 = call-poly <vilib>:"Delacor_lib_QMH_Enqueue Message (poly).vi"("Priority Message? (F)"=TRUE, "error in"=w479, "Message"="Exit", "Message Queue in"=w475) -> ("error out"=w476:errorcluster)  [unwired: 6 in, 1 out]
            n118 = Merge Errors(w476) -> (w477:errorcluster)
          }
          frame "Exit" {
            w485 = 91  # 91: not all Exit messages will have an argument
            w490 = TRUE  # Stop the VI
            # "Release the message queue reference"
            # "#CodeNeeded - Add any required cleanup code here"
            # "Exit - Exit the application."
            n119 = Variant To Data(error in=w494, type=T8 {"Origin"="", "Exit via Stop Module Req?"=FALSE, "Wait for Module to stop?"=FALSE} ("Stop Argument"), Variant=w487) -> (data=w483:T8, error out=w486:errorcluster)
            n120 = call <vilib>:"Clear Errors.vi"("error in (no error)"=w486, "specific error code to clear (0: all)"=w485) -> ("error out"=w493:errorcluster)  [unwired: 4 in, 1 out]
            n121 = call-dynamic "Delacor_lib_QMH_Release Message Queue.vi"("error in"=w493, "Message Queue"=w492) -> ("error out"=w489:errorcluster)  [unwired: 9 in]
            n122 = call "Sleep Ping Helper Loop.vi"() -> ("error out"=w480:errorcluster)  [unwired: 11 in]
            n123 = call "Handle Exit.vi"("Stop Argument"=w483, "Admin in"=w481) -> ("error out"=w482:errorcluster)  [unwired: 8 in, 1 out]
            n124 = Merge Errors(w480, w482, w489) -> (w488:errorcluster)
            n125 = call "Error Reported.vi"("Error"=w488) -> ()  [unwired: 10 in, 1 out]
          }
          frame Default {
            # "'Default' case only runs if there is a message that isn't defined in any of the other cases.  Output a programming error."
            n126 = call "Module Name--constant.vi"() -> ("Module Name"=w495:string)  [unwired: 11 in]
            n127 = xnode "Error Ring"("parameter 0"=w496, "parameter 1"=w495) -> ("error out"=w497:errorcluster)
          }
        }
        n128 = call-dynamic "Delacor_lib_QMH_Error Handler - Message Handling Loop.vi"("error in"=w245, "Message Queue in"=w236) -> ("dup error in"=w235:errorcluster)  [unwired: 8 in, 1 out]
      }
      n129 = while {
        tunnel: w45 -> [w84]
        shift-right: [w82] -> w48
        shift-left: w46 -> [w83]
        tunnel: [w78] -> w44
        tunnel: w42 -> [w77]
        tunnel: w41 -> [w76]
        shift-right: [w74] -> w39
        shift-left: w40 -> [w75]
        stop <- w80 stop-if-true
        # "Event Handling Loop"
        n130 = event "DQMH_EVENT_MAIN" shown="[13] <MQTTClient Request Events.Connect to MQTT Server>: User Event" {
          selector: w83 -> [_ _ _ _ _ _ _ _ _ _ _ _ _ _ _ _ _ w223 _]
          dyn-events: [_ _ _ _ _ _ _ _ _ _ _ _ _ _ _ _ _ w222 _] -> w82
          timeout: _ -> [_ _ _ _ _ _ _ _ _ _ _ _ _ _ _ _ _ _ _]
          tunnel: [_ _ _ _ _ _ TRUE ("Discard?") _ _ _ _ _ _ _ _ _ _ _ _] -> w80
          tunnel: w84 -> [w88 w100 w104 w107 w111 w116 w128 w138 w145 w164 w172 w181 w189 w197 w205 w213 w217 w225 w233]
          tunnel: [w87 w97 w102 _ w110 w113 w122 w134 w144 w155 w165 w173 w182 w190 w198 w207 w215 _ w226] -> w81
          tunnel: [w88 w99 w104 w107 w111 w115 w127 w138 w143 w162 w170 w179 w187 w195 w203 w211 w216 w225 w231] -> w79
          tunnel: w77 -> [_ _ _ _ _ _ _ _ w142 _ _ _ _ _ _ _ _ _ _]
          tunnel: w76 -> [_ _ _ _ _ _ _ w133 _ _ _ _ _ _ _ _ _ _ _]
          tunnel: w75 -> [w85 w96 w103 w106 w108 w112 w117 w137 w140 w163 w171 w180 w188 w196 w204 w212 w219 w224 w232]
          tunnel: [w85 w96 w103 w106 w108 w112 w117 w132 w139 w163 w171 w180 w188 w196 w204 w212 w219 w224 w232] -> w74
          event "Simulate EHL Error": Value Change {
            # "This case simulates an error being generated at the EHL"
            n131 = event-data() -> ()  [unwired: 1 in, 1 out]
            n132 = call "Module Name--constant.vi"() -> ("Module Name"=w86:string)  [unwired: 11 in]
            n133 = xnode "Error Ring"("parameter 0"=w86) -> ("error out"=w87:errorcluster)
          }
          event "Simulate MHL Error": Value Change {
            # "This case simulates an error being generated at the EHL"
            n134 = event-data() -> ()  [unwired: 1 in, 1 out]
            n135 = call-poly <vilib>:"Delacor_lib_QMH_Enqueue Message (poly).vi"("Message"="Simulate MHL Error", "Message Queue in"=w100) -> ("error out"=w97:errorcluster, "Message Queue out"=w99:refnum<class "Delacor_lib_QMH_Message Queue.lvclass">)  [unwired: 8 in]
          }
          event User Event {
            # "Another Module called the \"Show Panel\" API Method."
            n136 = event-data() -> ()  [unwired: 1 in, 1 out]
            n137 = call <vilib>:"Show.vi"("Panel in"=w103) -> ("Error Out"=w102:errorcluster)  [unwired: 10 in]
            n138 = call "Status Updated.vi"("Status"="Panel shown." ("format string")) -> ()  [unwired: 10 in, 1 out]
          }
          event User Event {
            # "Another Module called the \"Hide Panel\" API Method."
            n139 = event-data() -> ()  [unwired: 1 in, 1 out]
            n140 = call <vilib>:"Hide.vi"("Panel In"=w106) -> ()  [unwired: 10 in, 1 out]
            n141 = call "Status Updated.vi"("Status"="Panel hidden." ("format string")) -> ()  [unwired: 10 in, 1 out]
          }
          event User Event {
            # "Another Module called the \"Get Module Execution Status\" API Method."
            n142 = event-data() -> ()  [unwired: 1 in, 1 out]
            n143 = call "Update Module Execution Status.vi"("Running?"=TRUE) -> ("error out"=w110:errorcluster)  [unwired: 10 in]
          }
          event User Event {
            # "Another Module called the \"Show Diagram\" API Method."
            n144 = event-data() -> ()  [unwired: 1 in, 1 out]
            n145 = call-poly <vilib>:"Delacor_lib_QMH_Enqueue Message (poly).vi"("Message"="Show Diagram", "Message Queue in"=w116) -> ("error out"=w113:errorcluster, "Message Queue out"=w115:refnum<class "Delacor_lib_QMH_Message Queue.lvclass">)  [unwired: 8 in]
          }
          event User Event {
            # "The Stop Module Event can get fired from the Exit message in the MHL. The queue gets destroyed in that case. If the queue no longer exists, the Enqueue Exit as a priority message will return error 1. It is safe to ignore, because the module is already exiting."
            # "Another Module called the \"Stop Module\" API Method  or the Message Handling Loop below."
            n146 = event-data() -> ("Origin"=w126:string, "Exit via Stop Module Req?"=w120:bool, "Wait for Module to stop?"=w119:bool)  [unwired: 1 in]
            n147 = call <vilib>:"Hide.vi"("Panel In"=w117) -> ()  [unwired: 10 in, 1 out]
            n148 = local write "Status"(w126) -> ()
            n149 = Bundle By Name(cluster=T8 {"Origin"="", "Exit via Stop Module Req?"=FALSE, "Wait for Module to stop?"=FALSE} ("Stop Argument"), "Exit via Stop Module Req?"=w120, "Wait for Module to stop?"=w119) -> (w118:T8)
            n150 = call-poly <vilib>:"Delacor_lib_QMH_Enqueue Message (poly).vi"("Priority Message? (F)"=TRUE, "Message Data"=w118, "Message"="Exit", "Message Queue in"=w128) -> ("error out"=w123:errorcluster, "Message Queue out"=w127:refnum<class "Delacor_lib_QMH_Message Queue.lvclass">)  [unwired: 6 in]
            n151 = call <vilib>:"Clear Errors.vi"("error in (no error)"=w123, "specific error code to clear (0: all)"=1) -> ("error out"=w122:errorcluster)  [unwired: 4 in, 1 out]
          }
          event User Event {
            # "Another Module called the \"Change Panel\" API Method."
            n152 = event-data() -> ("New Panel"=w136:refnum<class "Panel.lvclass">)  [unwired: 1 in]
            n153 = call-dynamic <vilib>:"Close.vi"("Panel In"=w137) -> ("Error Out"=w135:errorcluster)  [unwired: 10 in]
            n154 = call <vilib>:"Initialize.vi"("error in (no error)"=w135, "My Helper in"=w133, "Panel In"=w136) -> ("error out"=w134:errorcluster, "Panel Out"=w132:refnum<class "Panel.lvclass">)  [unwired: 6 in, 1 out]
            n155 = call "Status Updated.vi"("Status"="Panel changed.") -> ()  [unwired: 10 in, 1 out]
          }
          event Panel Close? {
            w146 = TRUE  # Discard the event so the 'Confirm Quit' message has a chance to run.
            # "If launched externally, closing the panel doesn't quit the VI."
            # "Send the 'Confirm Quit' message if the user closes the panel of the VI."
            n156 = event-data() -> ()  [unwired: 1 in, 1 out]
            n157 = property class="Module Admin"(reference=w142) -> ("Accessors:External Launch"=w141:bool)  [unwired: 1 in, 2 out]
            n158 = case shown="True" w141 {
              tunnel: w145 -> [w151 w154]
              tunnel: [w150 w152] -> w144
              tunnel: [w149 w154] -> w143
              tunnel: w140 -> [w147 w153]
              tunnel: [w147 w153] -> w139
              frame False {
                n159 = call-poly <vilib>:"Delacor_lib_QMH_Enqueue Message (poly).vi"("Message"="Confirm Quit", "Message Queue in"=w151) -> ("error out"=w150:errorcluster, "Message Queue out"=w149:refnum<class "Delacor_lib_QMH_Message Queue.lvclass">)  [unwired: 8 in]
              }
              frame True {
                n160 = call <vilib>:"Hide.vi"("Panel In"=w153) -> ("Error Out"=w152:errorcluster)  [unwired: 10 in]
              }
            }
            n161 = event-data("Discard?"=w146) -> ()  [unwired: 1 in, 1 out]
          }
          event User Event {
            # "Another Module called the \"Initialise Connection\" API Method."
            n162 = event-data() -> ("Client ID"=w158:string, "Server Address"=w157:string, "Server Port"=w156:u16)  [unwired: 1 in]
            n163 = Bundle(cluster=T9 {"Client ID"="BTSCLIENT-001", "Server Address"="localhost", "Server Port"=1883} ("Initialise Connection Argument"), "Client ID"=w158, "Server Address"=w157, "Server Port"=w156) -> (w159:T9)
            n164 = call-poly <vilib>:"Delacor_lib_QMH_Enqueue Message (poly).vi"("Message Data"=w159, "Message"="Initialise Connection", "Message Queue in"=w164) -> ("error out"=w155:errorcluster, "Message Queue out"=w162:refnum<class "Delacor_lib_QMH_Message Queue.lvclass">)  [unwired: 7 in]
          }
          event User Event {
            # "Another Module called the \"Ping Connection\" API Method."
            n165 = event-data() -> ("Boolean"=w166:bool)  [unwired: 1 in]
            n166 = Bundle(cluster=T10 {"Boolean"=FALSE} ("Ping Connection Argument"), "Boolean"=w166) -> (w167:T10)
            n167 = call-poly <vilib>:"Delacor_lib_QMH_Enqueue Message (poly).vi"("Message Data"=w167, "Message"="Ping Connection", "Message Queue in"=w172) -> ("error out"=w165:errorcluster, "Message Queue out"=w170:refnum<class "Delacor_lib_QMH_Message Queue.lvclass">)  [unwired: 7 in]
          }
          event User Event {
            # "Another Module called the \"Publish to MQTT Topic\" API Method."
            n168 = event-data() -> ("Topic"=w175:string, "Value"=w174:string)  [unwired: 1 in]
            n169 = Bundle(cluster=T11 {"Topic"="", "Value"=""} ("Publish to MQTT Topic Argument"), "Topic"=w175, "Value"=w174) -> (w176:T11)
            n170 = call-poly <vilib>:"Delacor_lib_QMH_Enqueue Message (poly).vi"("Message Data"=w176, "Message"="Publish to MQTT Topic", "Message Queue in"=w181) -> ("error out"=w173:errorcluster, "Message Queue out"=w179:refnum<class "Delacor_lib_QMH_Message Queue.lvclass">)  [unwired: 7 in]
          }
          event User Event {
            # "Another Module called the \"Close Connection\" API Method."
            n171 = event-data() -> ("Boolean"=w183:bool)  [unwired: 1 in]
            n172 = Bundle(cluster=T12 {"Boolean"=FALSE} ("Close Connection Argument"), "Boolean"=w183) -> (w184:T12)
            n173 = call-poly <vilib>:"Delacor_lib_QMH_Enqueue Message (poly).vi"("Message Data"=w184, "Message"="Close Connection", "Message Queue in"=w189) -> ("error out"=w182:errorcluster, "Message Queue out"=w187:refnum<class "Delacor_lib_QMH_Message Queue.lvclass">)  [unwired: 7 in]
          }
          event User Event {
            # "Another Module called the \"Connect to MQTT Server\" API Method."
            n174 = event-data() -> ("Boolean"=w191:bool)  [unwired: 1 in]
            n175 = Bundle(cluster=T13 {"Boolean"=FALSE} ("Connect to MQTT Server Argument"), "Boolean"=w191) -> (w192:T13)
            n176 = call-poly <vilib>:"Delacor_lib_QMH_Enqueue Message (poly).vi"("Message Data"=w192, "Message"="Connect to MQTT Server", "Message Queue in"=w197) -> ("error out"=w190:errorcluster, "Message Queue out"=w195:refnum<class "Delacor_lib_QMH_Message Queue.lvclass">)  [unwired: 7 in]
          }
          event User Event {
            # "This module called the \"Private.Sleep Ping Helper Loop\" private request."
            n177 = event-data() -> ("Boolean"=w199:bool)  [unwired: 1 in]
            n178 = Bundle(cluster=T14 {"Boolean"=FALSE} ("Sleep Ping Helper Loop Argument"), "Boolean"=w199) -> (w200:T14)
            n179 = call-poly <vilib>:"Delacor_lib_QMH_Enqueue Message (poly).vi"("Message Data"=w200, "Message"="Sleep Ping Helper Loop", "Message Queue in"=w205) -> ("error out"=w198:errorcluster, "Message Queue out"=w203:refnum<class "Delacor_lib_QMH_Message Queue.lvclass">)  [unwired: 7 in]
          }
          event User Event {
            # "Another Module called the \"Subscribe to MQTT Topic\" API Method."
            n180 = event-data() -> ("Topic"=w206:string)  [unwired: 1 in, 4 out]
            n181 = Bundle(cluster=T15 {"Topic"=""} ("Subscribe to MQTT Topic Argument"), "Topic"=w206) -> (w208:T15)
            n182 = call-poly <vilib>:"Delacor_lib_QMH_Enqueue Message (poly).vi"("Message Data"=w208, "Message"="Subscribe to MQTT Topic", "Message Queue in"=w213) -> ("error out"=w207:errorcluster, "Message Queue out"=w211:refnum<class "Delacor_lib_QMH_Message Queue.lvclass">)  [unwired: 7 in]
          }
          event User Event {
            n183 = event-data() -> ("PUBLISH"=w214:refnum<class "PUBLISH.lvclass">)  [unwired: 1 in]
            n184 = call-poly <vilib>:"Delacor_lib_QMH_Enqueue Message (poly).vi"("Message Data"=w214, "Message"="Handle PUBLISH Data", "Message Queue in"=w217) -> ("error out"=w215:errorcluster, "Message Queue out"=w216:refnum<class "Delacor_lib_QMH_Message Queue.lvclass">)  [unwired: 7 in]
          }
          event User Event {
            n185 = event-data() -> ("Client Public Events"=w221:T1, "MQTT Public Events"=w220:T2)  [unwired: 1 in]
            n186 = register-events(reference=w223, w221, w220) -> (reference out=w222:refnum<event-registration>)  [unwired: 3 in, 1 out]
          }
          event User Event {
            # "Another Module called the \"Launch\" API Method."
            n187 = event-data() -> ("Boolean"=w227:bool)  [unwired: 1 in]
            n188 = Bundle(cluster=T16 {"Boolean"=FALSE} ("Launch Argument"), "Boolean"=w227) -> (w228:T16)
            n189 = call-poly <vilib>:"Delacor_lib_QMH_Enqueue Message (poly).vi"("Message Data"=w228, "Message"="Launch", "Message Queue in"=w233) -> ("error out"=w226:errorcluster, "Message Queue out"=w231:refnum<class "Delacor_lib_QMH_Message Queue.lvclass">)  [unwired: 7 in]
          }
        }
        n190 = call-dynamic "Delacor_lib_QMH_Error Handler - Event Handling Loop.vi"("error in"=w81, "Message Queue in"=w79) -> ("dup error in"=w78:errorcluster)  [unwired: 8 in, 1 out]
      }
      n191 = while {
        tunnel: w38 -> [w67]
        shift-right: [w65] -> _
        shift-left: -1 -> [w64]
        stop <- w66 stop-if-true
        # "Ping Helper Loop"
        n192 = event shown="[0] Timeout" {
          selector: w67 -> [_ _ _ _]
          dyn-events: _ -> [_ _ _ _]
          timeout: w64 -> [_ _ _ _]
          tunnel: [_ _ _ TRUE] -> w66
          tunnel: [w69 12000 -1 -1] -> w65
          tunnel: w64 -> [w69 _ _ _]
          tunnel: [w68 _ _ _] -> _
          event Timeout {
            n193 = event-data() -> ()  [unwired: 1 in, 3 out]
            n194 = call "Ping Connection.vi"() -> ("error out"=w68:errorcluster)  [unwired: 11 in]
          }
          event User Event {
            n195 = event-data() -> ()  [unwired: 1 in, 5 out]
          }
          event User Event {
            n196 = event-data() -> ()  [unwired: 1 in, 5 out]
          }
          event User Event {
            n197 = event-data() -> ()  [unwired: 1 in, 7 out]
          }
        }
      }
      n198 = while "DQMH_HELPER_LOOP" {
        shift-right: [w57] -> _
        shift-left: -1 -> [w56]
        shift-right: [w54] -> w35
        shift-left: w34 -> [w55]
        tunnel: w45 -> [w51]
        stop <- w53 stop-if-true
        w50 = "Connection Helper Loop"  # DQMH_HELPER_LOOP_NAME
        # "Connection Helper Loop"
        n199 = event "DQMH_HELPER_EVENT_STRUCTURE" shown="[0] Timeout" {
          selector: w55 -> [_ _ _]
          dyn-events: [_ _ _] -> w54
          timeout: w56 -> [_ _ _]
          tunnel: w56 -> [_ w62 _]
          tunnel: [-1 w62 1000] -> w57
          tunnel: [_ TRUE _] -> w53
          tunnel: [w58 errorcluster {"status"=FALSE, "code"=0, "source"=""} ("error constant") _] -> w52
          tunnel: w51 -> [_ _ _]
          event Timeout {
            n200 = event-data() -> ()  [unwired: 1 in, 1 out]
            n201 = call "Connect to MQTT Server.vi"() -> ("error out"=w58:errorcluster)  [unwired: 11 in]
          }
          event User Event {
            n202 = event-data() -> ()  [unwired: 1 in, 1 out]
          }
          event User Event {
            # "This module called the \"Private.Wake Connection Helper Loop\" private request."
            n203 = event-data() -> ()  [unwired: 1 in, 1 out]
          }
        }
        n204 = call-dynamic "Delacor_lib_QMH_Error Handler - Helper Loop.vi"("Error Debug"=w50, "error in"=w52, "Message Queue in"=w51) -> ()  [unwired: 7 in, 2 out]
      }
      n205 = Unregister For Events(event registration refnum=w35) -> ()  [unwired: 1 in, 1 out]
    }
    frame Error {
      # "Synchronize Caller Events.vi will inform Start Module.vi that the module has launched and will let the code calling Start Module.vi register for broadcasts and would permit the caller receive the broadcast that an error occurred at launch time."
      n206 = call-dynamic "Delacor_lib_QMH_Release Message Queue.vi"("Message Queue"=w507) -> ()  [unwired: 10 in, 1 out]
      n207 = call "Synchronize Caller Events.vi"("Singleton Module Admin in"=w512) -> ("error out"=w509:errorcluster)  [unwired: 9 in, 1 out]
      n208 = call "Module Name--constant.vi"() -> ("Module Name"=w515:string)  [unwired: 11 in]
      n209 = Format Into String(format string="An error occurred during initialization. %s is no longer running.", w515) -> (resulting string=w513:string)  [unwired: 2 in, 1 out]
      n210 = Merge Errors(w511, w509) -> (w510:errorcluster)
      n211 = call "Error Reported.vi"("Additional Information"=w513, "Error"=w510) -> ()  [unwired: 9 in, 1 out]
    }
  }
  n212 = Merge Errors(w24, w31) -> (w23:errorcluster)
  n213 = call "Close Module.vi"("error in (no error)"=w23, "Module Admin in"=w32) -> ("error out"=w26:errorcluster, "External Launch"=w21:bool, "Module Admin out"=w25:refnum<class "Delacor_lib_QMH_Module Admin.lvclass">)  [unwired: 7 in]
  n214 = Unregister For Events(event registration refnum=w30, error in=w26) -> (error out=w22:errorcluster)
  "error out" <- w22
  n215 = case "External Launch?" shown="True" w21 {
    tunnel: w22 -> [_ w521]
    tunnel: w19 -> [_ w520]
    tunnel: w11 -> [_ w518]
    frame False {
    }
    frame True {
      n216 = call-dynamic <vilib>:"Close.vi"("Panel In"=w520) -> ("Error Out"=w519:errorcluster)  [unwired: 10 in]
      n217 = call <vilib>:"Close.vi"("error in (no error)"=w519, "Controller in"=w518) -> ("error out"=w517:errorcluster)  [unwired: 9 in]
      n218 = case shown="Error" w521 {
        tunnel: w517 -> [_ _]
        frame No Error {
        }
        frame Error {
          n219 = disable-structure shown="Default" {
            frame condition #0 (active) {
              n220 = invoke class="VI" method="FP.Open"("Activate"=TRUE ("Activate?")) -> ()  [unwired: 4 in, 5 out]
            }
            frame condition #1 {
              # "Don't show panel on error if running inside a built EXE."
            }
          }
        }
      }
    }
  }
  n221 = local write "Module Admin"(w25) -> ()
